vi "Read SMU.vi"(8 "error in (no error)":errorcluster, 10 "Instruments in":T1, 11 "Use second SMUs":bool) -> (0 "error out":errorcluster, 3 "Instruments out":T1)   [LabVIEW 2021]
doc: "Reads actual measured value from single or both SMU. Adds a timestamp when readings are queried from SMU's."
uses:
  <instrlib>/Keithley 2450/Keithley 2450.lvlib
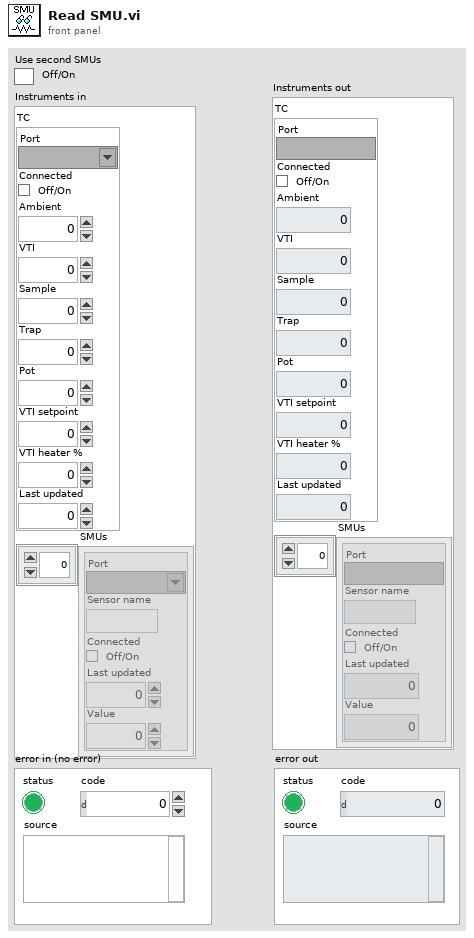
[diagram p1: front panel]
types:
  T1 = cluster{"TC":cluster{"Port":refnum<visa-resource-name>, "Connected":bool, "Ambient":dbl, "VTI":dbl, "Sample":dbl, "Trap":dbl, "Pot":dbl, "VTI setpoint":dbl, "VTI heater %":dbl, "Last updated":dbl}, "SMUs":cluster{"Port":refnum<visa-resource-name>, "Sensor name":string, "Connected":bool, "Last updated":dbl, "Value":dbl}[]}
  T2 = cluster{"Port":refnum<visa-resource-name>, "Sensor name":string, "Connected":bool, "Last updated":dbl, "Value":dbl}[]
  T3 = cluster{"Port":refnum<visa-resource-name>, "Sensor name":string, "Connected":bool, "Last updated":dbl, "Value":dbl}
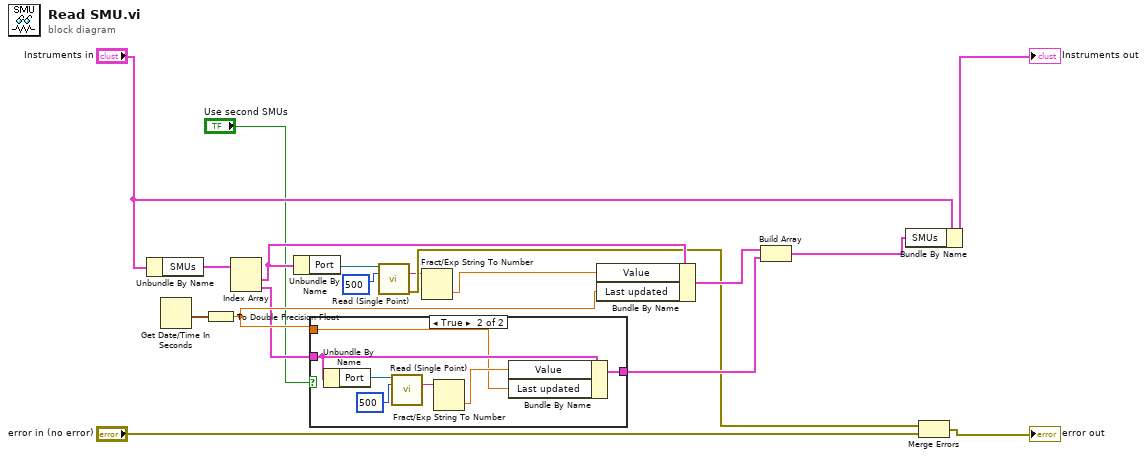
[diagram p0: block diagram]
diagram:
  n1 = Unbundle By Name("Instruments in") -> ("SMUs"=w2:T2)
  n2 = Get Date/Time In Seconds() -> (seconds since 1Jan1904=w15:timestamp)
  n3 = To Double Precision Float(number=w15) -> (double precision float=w16:dbl)
  n4 = Index Array(array=w2) -> (element #1=w12:T3, element #2=w5:T3)  [unwired: 2 in]
  n5 = Unbundle By Name(w12) -> ("Port"=w4:refnum<visa-resource-name>)
  n6 = case shown="True" "Use second SMUs" {
    tunnel: w5 -> [w19 w23]
    tunnel: [w19 w21] -> w10
    tunnel: w16 -> [_ w20]
    frame False {
    }
    frame True {
      n7 = Unbundle By Name(w23) -> ("Port"=w25:refnum<visa-resource-name>)
      n8 = call <instrlib>:"Read (Single Point).vi"("VISA resource name"=w25, "Timeout (10000 ms)"=500) -> ("Data out"=w26:string)  [unwired: 11 in, 2 out]
      n9 = Fract/Exp String To Number(string=w26) -> (number=w22:dbl)  [unwired: 3 in, 1 out]
      n10 = Bundle By Name(cluster=w23, "Value"=w22, "Last updated"=w20) -> (w21:T3)
    }
  }
  n11 = call <instrlib>:"Read (Single Point).vi"("VISA resource name"=w4, "Timeout (10000 ms)"=500) -> ("Data out"=w3:string, "error out"=w8:errorcluster)  [unwired: 11 in, 1 out]
  n12 = Fract/Exp String To Number(string=w3) -> (number=w11:dbl)  [unwired: 3 in, 1 out]
  n13 = Bundle By Name(cluster=w12, "Value"=w11, "Last updated"=w16) -> (w14:T3)
  n14 = Build Array(w14, w10) -> (w13:T2)
  n15 = Bundle By Name(cluster="Instruments in", "SMUs"=w13) -> (→"Instruments out":T1)
  n16 = Merge Errors(w8, "error in (no error)") -> (→"error out":errorcluster)
